vi "AnalyseSource.vi"(8 "error in (no error)":errorcluster, 11 "AllData In":T4 {"FlukeData"."DataAnalysisArray"."TimeStamp" format="%^<%.3X\n%x>T"; "FlukeData"."ModelDataArray"."FREQUENCY" format="%#_6f"; "FlukeData"."ModelDataArray"."TimeStamp" format="%^<%.3X\n%x>T"; "FlukeData"."PMUDataArray"."FREQUENCY" format="%#_6f"; "FlukeData"."PMUDataArray"."TimeStamp" format="%^<%.3X\n%x>T"; "NISTData"."DataAnlysisArray"."TimeStamp" format="%^<%.3X\n%x>T"; "NISTData"."DUTDataArray"."Time Stamp" format="%^<%.3X\n%x>T"; "NISTData"."NIDataArray"."Time Stamp" format="%^<%.3X\n%x>T"}) -> (0 "error out":errorcluster, 2 "ResultArray":T1 {"Time Stamp" format="%^<%.3X\n%x>T"}, 3 "AllData Out":T4 {"FlukeData"."DataAnalysisArray"."TimeStamp" format="%^<%.3X\n%x>T"; "FlukeData"."ModelDataArray"."FREQUENCY" format="%#_6f"; "FlukeData"."ModelDataArray"."TimeStamp" format="%^<%.3X\n%x>T"; "FlukeData"."PMUDataArray"."FREQUENCY" format="%#_6f"; "FlukeData"."PMUDataArray"."TimeStamp" format="%^<%.3X\n%x>T"; "NISTData"."DataAnlysisArray"."TimeStamp" format="%^<%.3X\n%x>T"; "NISTData"."DUTDataArray"."Time Stamp" format="%^<%.3X\n%x>T"; "NISTData"."NIDataArray"."Time Stamp" format="%^<%.3X\n%x>T"})   [LabVIEW 2014]
uses:
  typedefs/Alldata.ctl
  typedefs/NISTData.ctl
  typedefs/NIDataArray.ctl
  typedefs/NIData.ctl
  typedefs/PhasorRectangular.ctl
  typedefs/DUTData.ctl
  typedefs/NICalcAnalysis.ctl
  typedefs/CalcPhasorError.ctl
  typedefs/PlotDataArrays.ctl
  typedefs/PmuRawDataCluster.ctl
  typedefs/CalcAnalysis.ctl
  typedefs/ResultArray.ctl
  typedefs/Result.ctl
  typedefs/TVE_Fe_RFE.ctl
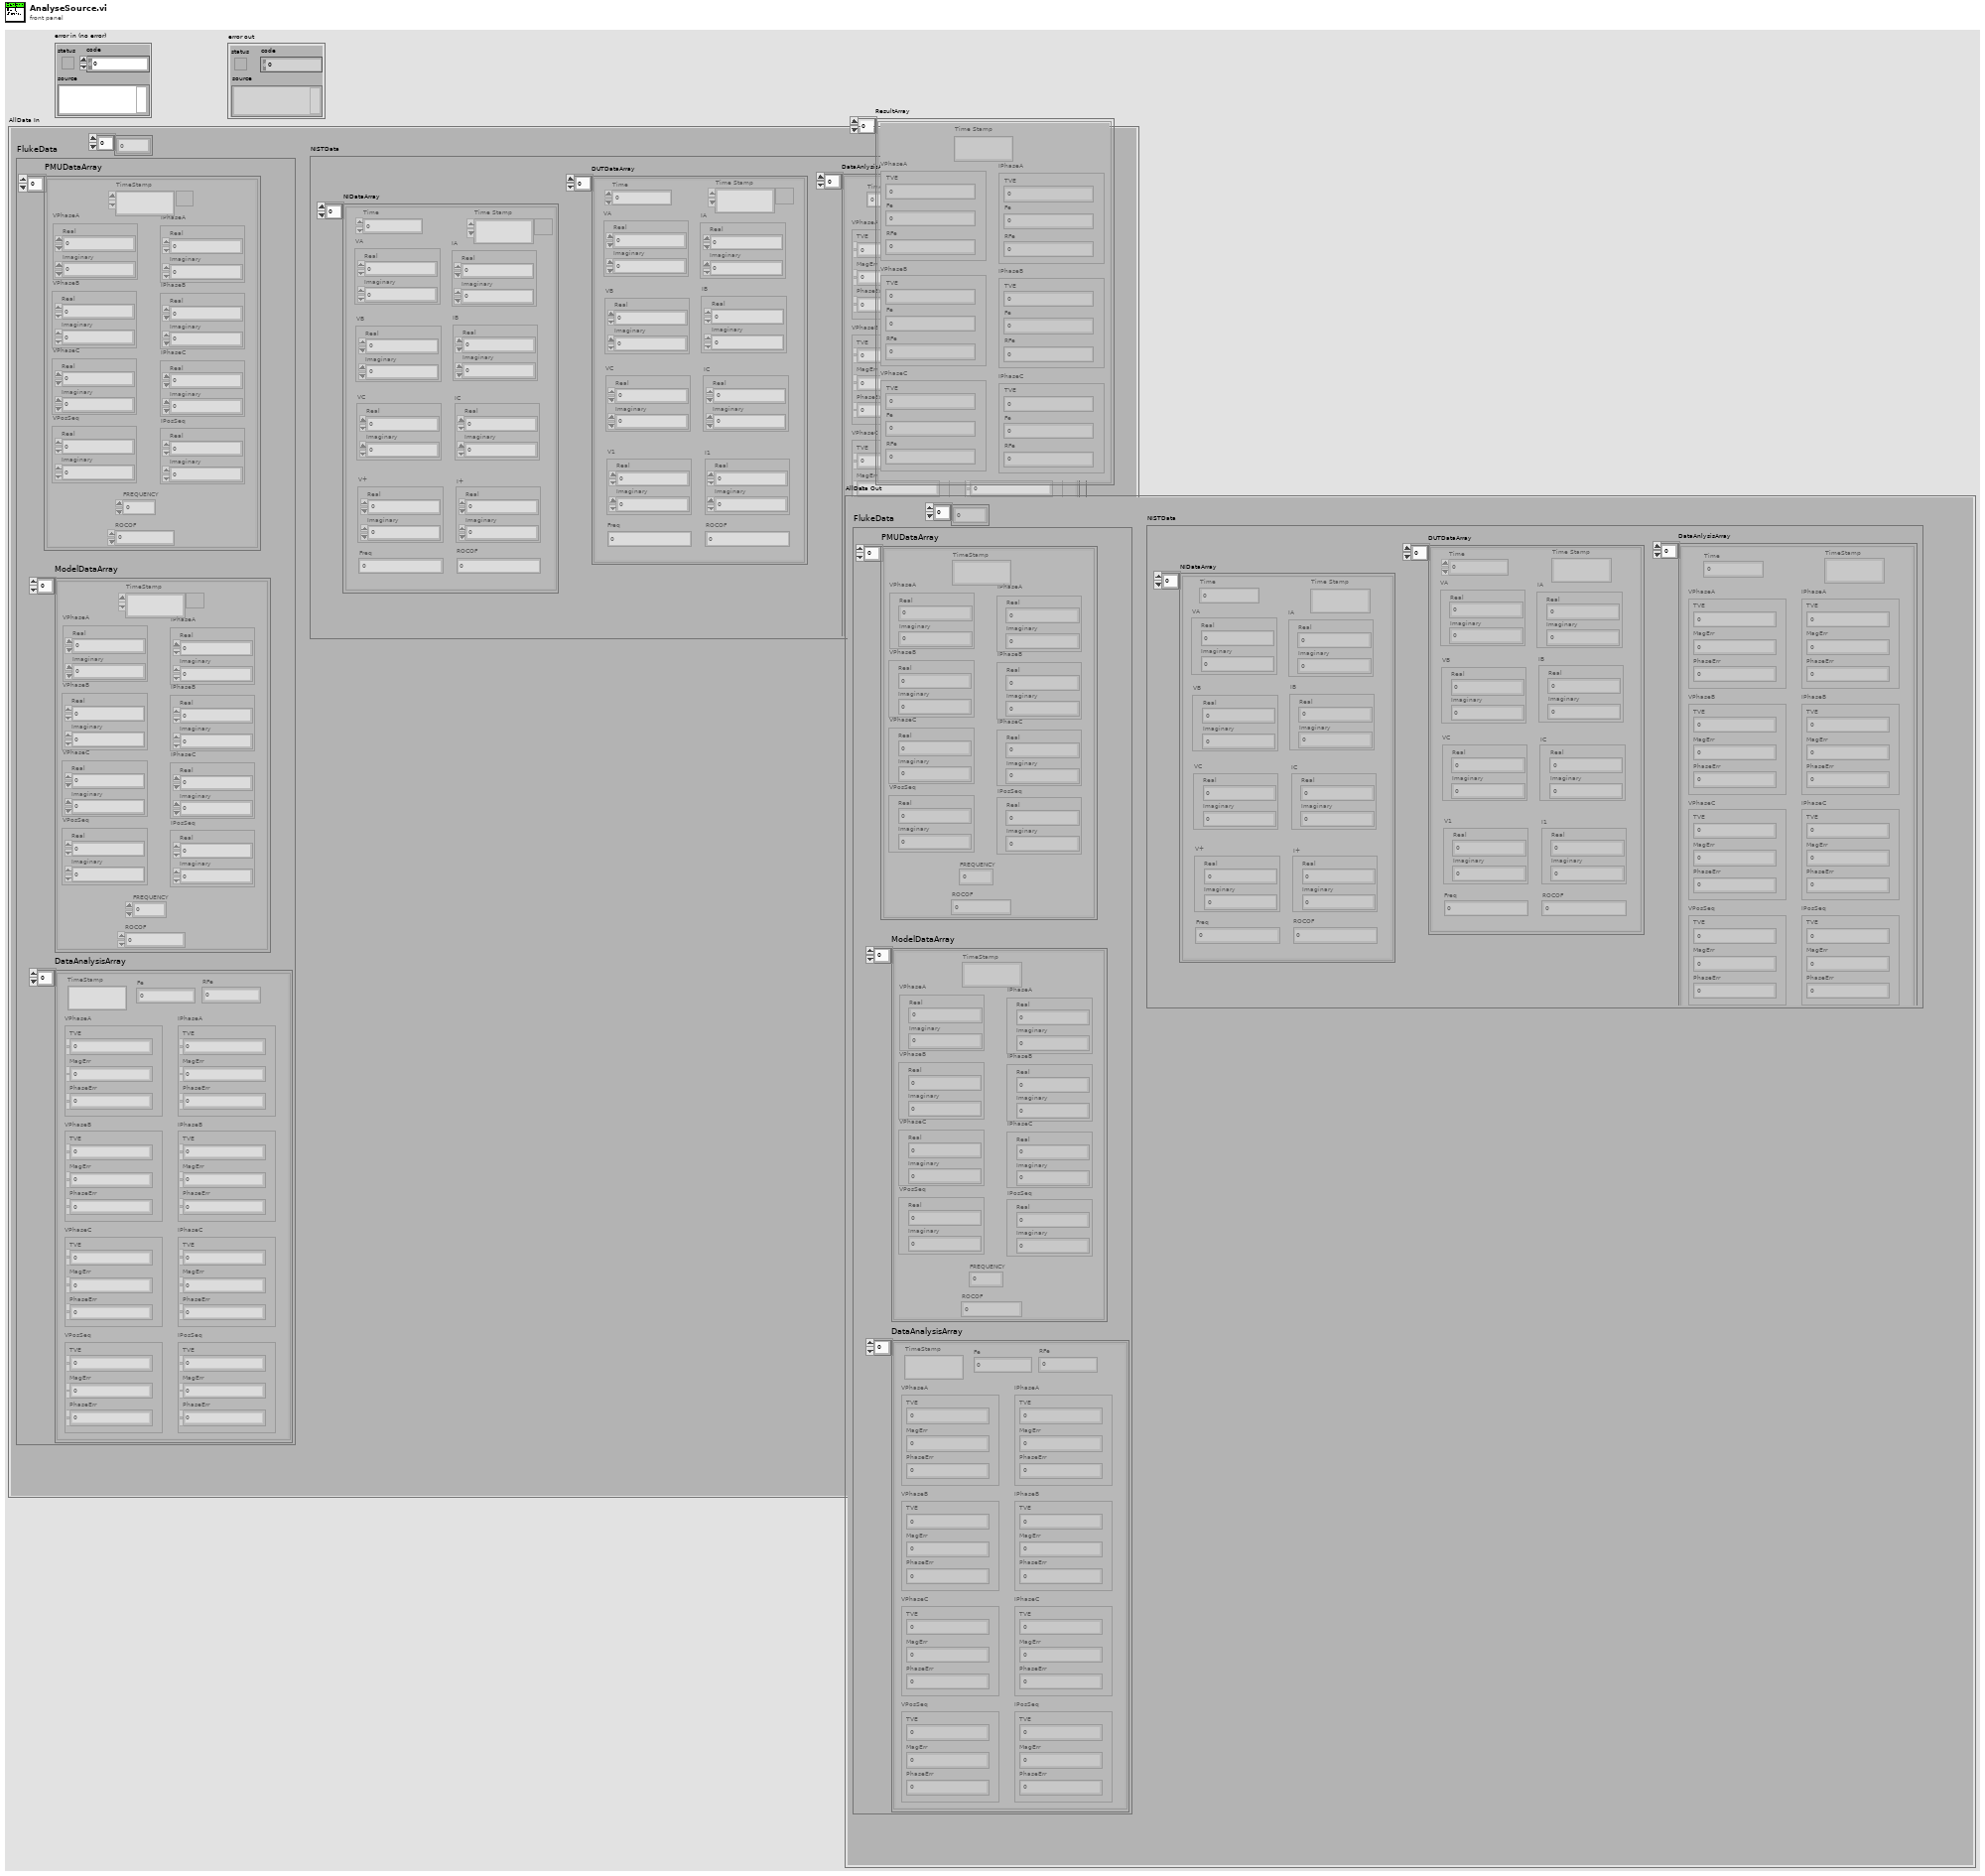
[diagram p1: front panel]
types:
  T1 = typedef "ResultArray.ctl" = T2[]
  T2 = typedef "Result.ctl" = cluster{"Time Stamp":timestamp, "VPhaseA":T3, "VPhaseB":T3, "VPhaseC":T3, "IPhaseA":T3, "IPhaseB":T3, "IPhaseC":T3}
  T3 = typedef "TVE_Fe_RFE.ctl" = cluster{"TVE":dbl, "Fe":dbl, "RFe":dbl}
  T4 = typedef "Alldata.ctl" = cluster{"NISTData":T5, "FlukeData":T12, "Params":dbl[]}
  T5 = typedef "NISTData.ctl" = cluster{"NIDataArray":T6, "DUTDataArray":T9[], "DataAnlysisArray":T10[]}
  T6 = typedef "NIDataArray.ctl" = T7[]
  T7 = typedef "NIData.ctl" = cluster{"Time":dbl, "VA":T8, "VB":T8, "VC":T8, "V+":T8, "IA":T8, "IB":T8, "IC":T8, "I+":T8, "Freq":dbl, "ROCOF":dbl, "Time Stamp":timestamp}
  T8 = typedef "PhasorRectangular.ctl" = cluster{"Real":dbl, "Imaginary":dbl}
  T9 = typedef "DUTData.ctl" = cluster{"Time":dbl, "VA":T8, "VB":T8, "VC":T8, "V1":T8, "IA":T8, "IB":T8, "IC":T8, "I1":T8, "Freq":dbl, "ROCOF":dbl, "Time Stamp":timestamp}
  T10 = typedef "NICalcAnalysis.ctl" = cluster{"Time":dbl, "VPhaseA":T11, "IPhaseA":T11, "VPhaseB":T11, "IPhaseB":T11, "VPhaseC":T11, "IPhaseC":T11, "VPosSeq":T11, "IPosSeq":T11, "Fe":dbl, "RFe":dbl, "TimeStamp":timestamp}
  T11 = typedef "CalcPhasorError.ctl" = cluster{"TVE":dbl, "MagErr":dbl, "PhaseErr":dbl}
  T12 = typedef "PlotDataArrays.ctl" = cluster{"PMUDataArray":T13[], "ModelDataArray":T13[], "DataAnalysisArray":T14[]}
  T13 = typedef "PmuRawDataCluster.ctl" = cluster{"TimeStamp":timestamp, "VPhaseA":T8, "VPhaseB":T8, "VPhaseC":T8, "VPosSeq":T8, "IPhaseA":T8, "IPhaseB":T8, "IPhaseC":T8, "IPosSeq":T8, "FREQUENCY":dbl, "ROCOF":sgl}
  T14 = typedef "CalcAnalysis.ctl" = cluster{"TimeStamp":timestamp, "VPhaseA":T11, "VPhaseB":T11, "VPhaseC":T11, "VPosSeq":T11, "IPhaseA":T11, "IPhaseB":T11, "IPhaseC":T11, "IPosSeq":T11, "Fe":dbl, "RFe":dbl}
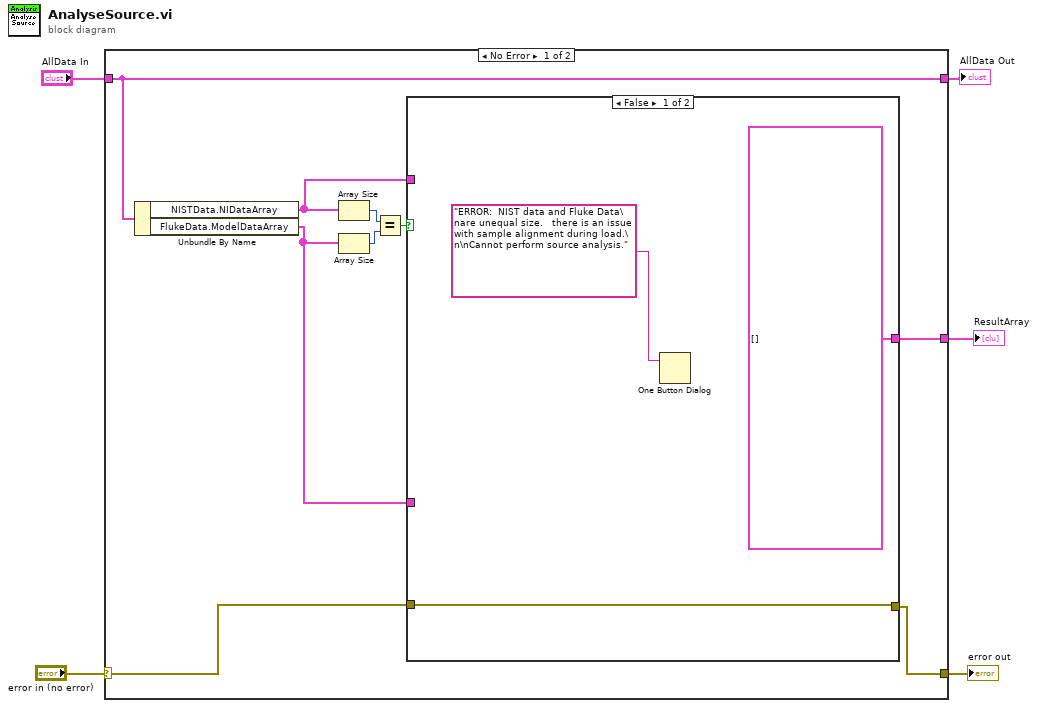
[diagram p0: block diagram]
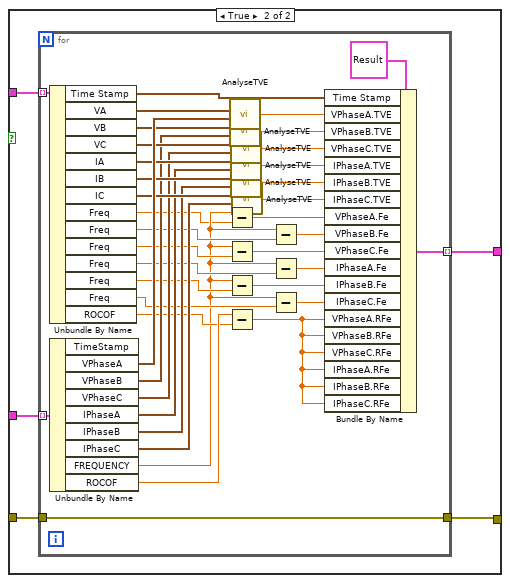
[diagram p2: hidden frame]
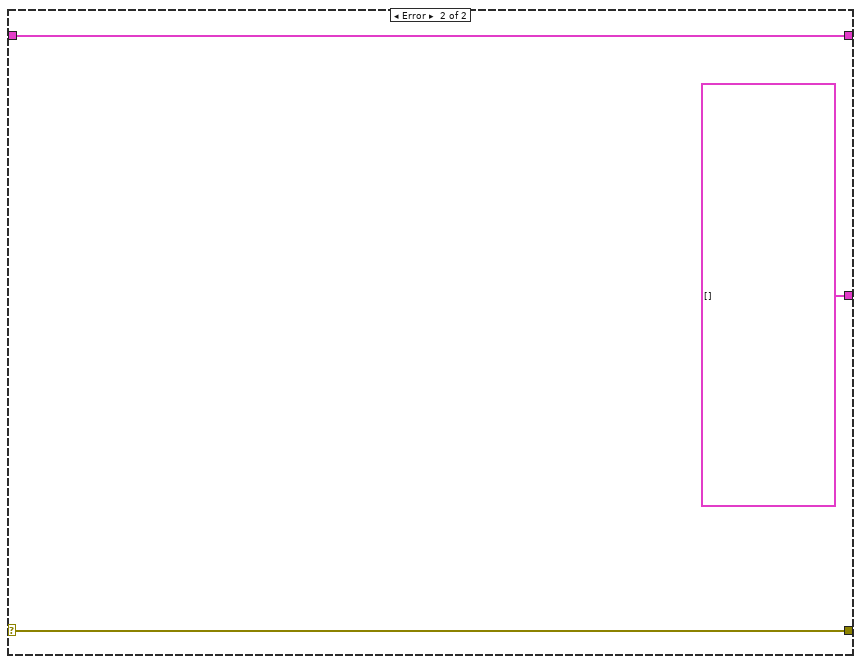
[diagram p3: hidden frame]
diagram:
  n1 = case shown="No Error" "error in (no error)" {
    selector: "error in (no error)" -> [w8 w64]
    tunnel: [w14 w65] -> w4
    tunnel: "AllData In" -> [w14 w65]
    tunnel: [w7 T2[] []] -> w2
    tunnel: [w6 w64] -> w1
    frame No Error {
      n2 = Unbundle By Name(w14) -> ("NISTData.NIDataArray"=w13:T6, "FlukeData.ModelDataArray"=w12:T13[])
      n3 = Array Size(array=w13) -> (size(s)=w10:i32)
      n4 = Array Size(array=w12) -> (size(s)=w11:i32)
      n5 = Equal?(x=w10, y=w11) -> (x = y?=w9:bool)
      n6 = case shown="False" w9 {
        tunnel: w13 -> [_ w22]
        tunnel: w12 -> [_ w21]
        tunnel: w8 -> [w16 w20]
        tunnel: [T2[] [] w19] -> w7
        tunnel: [w16 w18] -> w6
        frame False {
          n7 = One Button Dialog(message="ERROR:  NIST data and Fluke Data\nare unequal size.   there is an issue with sample alignment during load.\n\nCannot perform source analysis.") -> ()  [unwired: 1 in, 1 out]
        }
        frame True {
          n8 = for {
            tunnel: w22 -> [w62] mode=indexing
            tunnel: w21 -> [w61] mode=indexing
            tunnel: w20 -> [w32]
            tunnel: [w33] -> w19 mode=indexing
            tunnel: [w32] -> w18
            n9 = Unbundle By Name(w62) -> ("Time Stamp"=w48:timestamp, "VA"=w60:T8, "VB"=w58:T8, "VC"=w57:T8, "IA"=w56:T8, "IB"=w55:T8, "IC"=w54:T8, "Freq"=w23:dbl, "Freq"=w25:dbl, "Freq"=w26:dbl, "Freq"=w27:dbl, "Freq"=w28:dbl, "Freq"=w29:dbl, "ROCOF"=w30:dbl)
            n10 = Unbundle By Name(w61) -> ("VPhaseA"=w59:T8, "VPhaseB"=w53:T8, "VPhaseC"=w52:T8, "IPhaseA"=w51:T8, "IPhaseB"=w50:T8, "IPhaseC"=w49:T8, "FREQUENCY"=w24:dbl, "ROCOF"=w31:sgl)  [unwired: 1 out]
            n11 = Subtract(x=w24, y=w23) -> (x-y=w41:dbl)
            n12 = Subtract(x=w24, y=w26) -> (x-y=w39:dbl)
            n13 = Subtract(x=w24, y=w28) -> (x-y=w37:dbl)
            n14 = Subtract(x=w31, y=w30) -> (x-y=w35:dbl)
            n15 = call "AnalyseTVE.vi"("NISTPhasor"=w60, "FlukePhasor"=w59) -> ("TVE"=w47:dbl)  [unwired: 5 in]
            n16 = call "AnalyseTVE.vi"("NISTPhasor"=w58, "FlukePhasor"=w53) -> ("TVE"=w46:dbl)  [unwired: 5 in]
            n17 = call "AnalyseTVE.vi"("NISTPhasor"=w57, "FlukePhasor"=w52) -> ("TVE"=w45:dbl)  [unwired: 5 in]
            n18 = call "AnalyseTVE.vi"("NISTPhasor"=w56, "FlukePhasor"=w51) -> ("TVE"=w44:dbl)  [unwired: 5 in]
            n19 = call "AnalyseTVE.vi"("NISTPhasor"=w55, "FlukePhasor"=w50) -> ("TVE"=w43:dbl)  [unwired: 5 in]
            n20 = call "AnalyseTVE.vi"("NISTPhasor"=w54, "FlukePhasor"=w49) -> ("TVE"=w42:dbl)  [unwired: 5 in]
            n21 = Subtract(x=w24, y=w25) -> (x-y=w40:dbl)
            n22 = Subtract(x=w24, y=w27) -> (x-y=w38:dbl)
            n23 = Subtract(x=w24, y=w29) -> (x-y=w36:dbl)
            n24 = Bundle By Name(cluster=T2 {"Time Stamp"=timestamp(0 s since 1904-01-01), "VPhaseA"={"TVE"=0.0, "Fe"=0.0, "RFe"=0.0}, "VPhaseB"={"TVE"=0.0, "Fe"=0.0, "RFe"=0.0}, "VPhaseC"={"TVE"=0.0, "Fe"=0.0, "RFe"=0.0}, "IPhaseA"={"TVE"=0.0, "Fe"=0.0, "RFe"=0.0}, "IPhaseB"={"TVE"=0.0, "Fe"=0.0, "RFe"=0.0}, "IPhaseC"={"TVE"=0.0, "Fe"=0.0, "RFe"=0.0}} ("Result"), "Time Stamp"=w48, "VPhaseA.TVE"=w47, "VPhaseB.TVE"=w46, "VPhaseC.TVE"=w45, "IPhaseA.TVE"=w44, "IPhaseB.TVE"=w43, "IPhaseC.TVE"=w42, "VPhaseA.Fe"=w41, "VPhaseB.Fe"=w40, "VPhaseC.Fe"=w39, "IPhaseA.Fe"=w38, "IPhaseB.Fe"=w37, "IPhaseC.Fe"=w36, "VPhaseA.RFe"=w35, "VPhaseB.RFe"=w35, "VPhaseC.RFe"=w35, "IPhaseA.RFe"=w35, "IPhaseB.RFe"=w35, "IPhaseC.RFe"=w35) -> (w33:T2)
          }
        }
      }
    }
    frame Error {
    }
  }
  "AllData Out" <- w4
  "error out" <- w1
  "ResultArray" <- w2
